vi "Autonomous Independent.vi"   [LabVIEW 2019]
doc: "This VI is called when autonomous begins, and will automatically be terminated when autonomous ends. You can carry out timed or sensor driven robot movement independently without needing to return to the caller."
uses:
  <vilib>/Rock Robotics/Network Tables/NT Read String.vi
panel:
  # "Be sure to right-click and choose Data Operations>>Make Current Value default if you want to save the array values with the VI"
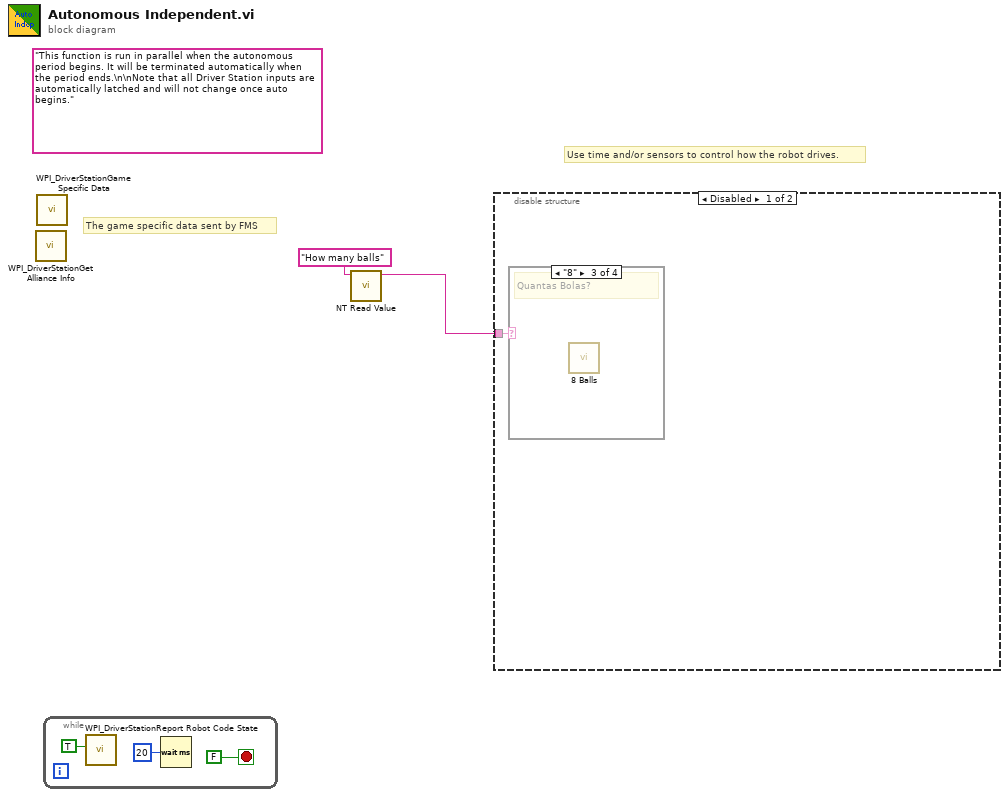
[diagram p0: block diagram]
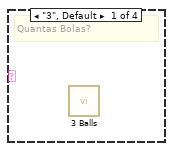
[diagram p2: hidden frame]
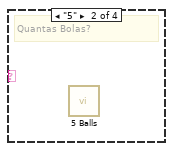
[diagram p3: hidden frame]
diagram:
  (unwired) "This function is run in parallel when the autonomous period begins. It will be terminated automatically when the period ends.\n\nNote that all Driver Station inputs are automatically latched and will not change once auto begins."
  # "The game specific data sent by FMS"
  # "Use time and/or sensors to control how the robot drives."
  n1 = call <vilib>:"WPI_DriverStationGet Alliance Info.vi"() -> ()  [unwired: 12 out]
  n2 = call <vilib>:"WPI_DriverStationGame Specific Data.vi"() -> ()  [unwired: 11 in, 1 out]
  n3 = while {
    stop <- FALSE stop-if-true
    n4 = call <vilib>:"WPI_DriverStationReport Robot Code State.vi"("Autonomous"=TRUE) -> ()  [unwired: 10 in, 1 out]
    n5 = Wait (ms)(milliseconds to wait=u32 20) -> ()  [unwired: 1 out]
  }
  n6 = call-poly <vilib>:"NT Read Value.vi"("Name"="How many balls") -> ("String"=w1:string)  [unwired: 9 in, 1 out]
  n7 = disable-structure shown="Disabled" {
    disable-tunnel: w1 -> [w6 _]
    frame Disabled {
      n8 = case shown="\"8\"" w6 {
        frame "3", Default {
          # "Quantas Bolas?"
          n9 = call "3 Balls.vi"() -> ()  [unwired: 12 in]
        }
        frame "5" {
          # "Quantas Bolas?"
          n10 = call "5 Balls.vi"() -> ()  [unwired: 12 in]
        }
        frame "8" {
          # "Quantas Bolas?"
          n11 = call "8 Balls.vi"() -> ()  [unwired: 12 in]
        }
        frame "10" {
        }
      }
    }
    frame Enabled {
    }
  }
